vi "StatusHistory Example.vi"() -> ()   [LabVIEW 2015]
doc: "This QControl modifies a string control to display a running status history to the user. Colors are used to match the string background to give a fade-out effect.\n\n1. Click Run.\n2. Every one second an item is added to the history.\n3. Change Options to see different configurations.\n (Normally these would be set on initialize and not change. However, \n they are changable at run-time.)\n4. Click Stop to end program.\n<b> </b> <b> </b>\n©2016 Q Software Innovations, LLC (QSI)\nwritten by Quentin Alldredge\nproduced in LabVIEW 2015\n\nsupport@qsoftwareinnovations.com\nwww.qsoftwareinnovations.com\n\nAll rights reserved.\n\nRedistribution and use in source and binary forms, with or without modification, are permitted provided that the following conditions are met:\n\n * Redistributions of source code must retain the above copyright notice, this list of conditions and the following disclaimer.\n * Redistributions in binary form must reproduce the above copyright notice, this list of conditions and the following disclaimer in the documentation and/or other materials provided with the distribution.\n * Neither the name of Q Software Innovations, LLC. nor the names of its contributors may be used to endorse or promote products derived from this software without specific prior written permission.\n\nTHIS SOFTWARE IS PROVIDED BY THE COPYRIGHT HOLDERS AND CONTRIBUTORS \"AS IS\" AND ANY EXPRESS OR IMPLIED WARRANTIES, INCLUDING, BUT NOT LIMITED TO, THE IMPLIED WARRANTIES OF MERCHANTABILITY AND FITNESS FOR A PARTICULAR PURPOSE ARE DISCLAIMED. IN NO EVENT SHALL THE COPYRIGHT OWNER OR CONTRIBUTORS BE LIABLE FOR ANY DIRECT, INDIRECT, INCIDENTAL, SPECIAL, EXEMPLARY, OR CONSEQUENTIAL DAMAGES (INCLUDING, BUT NOT LIMITED TO, PROCUREMENT OF SUBSTITUTE GOODS OR SERVICES; LOSS OF USE, DATA, OR PROFITS; OR BUSINESS INTERRUPTION) HOWEVER CAUSED AND ON ANY THEORY OF LIABILITY, WHETHER IN CONTRACT, STRICT LIABILITY, OR TORT (INCLUDING NEGLIGENCE OR OTHERWISE) ARISING IN ANY WAY OUT OF THE USE OF THIS SOFTWARE, EVEN IF ADVISED OF THE POSSIBILITY OF SUCH DAMAGE."
uses:
  QControl Classes/StatusHistory/StatusHistory.lvclass
  QControl Classes/StatusHistory/Direction.ctl
panel:
  in  "Most Recent Color":u32(colorbox)
  in  "Least Recent Color":u32(colorbox)
  in  "History Size":u32=1 caption="History Size (1-10)" min=1 max=10 step=1
  in  "Direction":T1
  in  "Stop Button":bool
  in  "StatusHistory":string
  # "StatusHistory QControl Example\n\nThis QControl modifies a string control to display a running status history to the user.  Colors are used to match the string background to give a fade-out effect.\n\n1. Click Run.\n2. Every one second an item is added to the history.\n3. Change Options to see different configurations.\n    (Normally these would be set on initialize and not change.  However, \n     they are changable at run-time.)\n4. Click Stop to end program."
  # "Options"
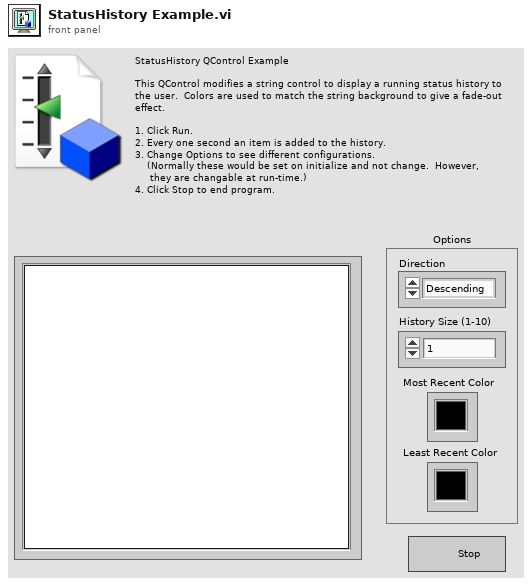
[diagram p1: front panel]
types:
  T1 = typedef "StatusHistory.lvclass/Direction.ctl" = enum16{"Descending", "Ascending"}
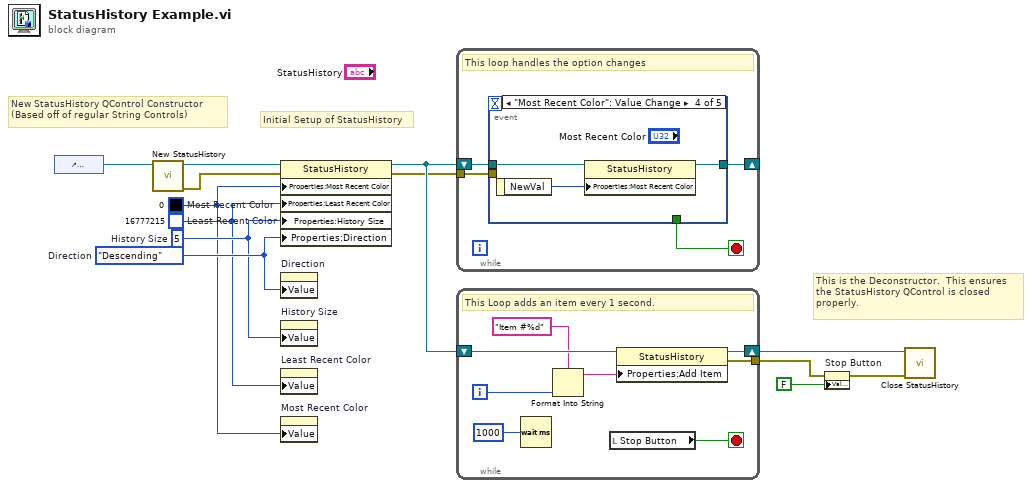
[diagram p0: block diagram]
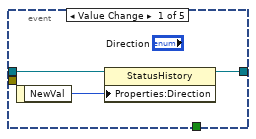
[diagram p2: hidden frame]
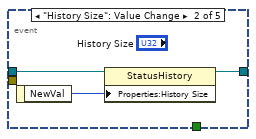
[diagram p3: hidden frame]
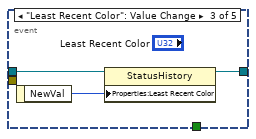
[diagram p4: hidden frame]
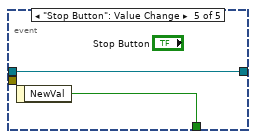
[diagram p5: hidden frame]
diagram:
  w7 = Direction."Descending"  # Direction
  w2 = u32 16777215  # Least Recent Color
  w1 = u32 0  # Most Recent Color
  w6 = u32 5  # History Size
  # "This is the Deconstructor.  This ensures \nthe StatusHistory QControl is closed \nproperly."
  # "Initial Setup of StatusHistory"
  # "New StatusHistory QControl Constructor\n(Based off of regular String Controls)"
  n1 = control-ref of="StatusHistory"() -> (w13:refnum<vi>)
  n2 = call "New StatusHistory.vi"("Reference"=w13) -> ("error out"=w11:errorcluster, "StatusHistory out"=w12:refnum<class "StatusHistory.lvclass">)  [unwired: 9 in]
  n3 = property class="StatusHistory"(reference=w12, error in=w11, "Properties:Most Recent Color"=w1, "Properties:Least Recent Color"=w2, "Properties:History Size"=w6, "Properties:Direction"=w7) -> (reference out=w10:refnum<class "StatusHistory.lvclass">, error out=w5:errorcluster)
  n4 = property on="Direction" class="Enum (strict)"("Value"=w7) -> ()  [unwired: 2 in, 2 out]
  n5 = property on="History Size" class="DigNum (strict)"("Value"=w6) -> ()  [unwired: 2 in, 2 out]
  n6 = property on="Least Recent Color" class="ColBox"("Value"=w2) -> ()  [unwired: 2 in, 2 out]
  n7 = property on="Most Recent Color" class="ColBox"("Value"=w1) -> ()  [unwired: 2 in, 2 out]
  n8 = while {
    shift-right: [w16] -> _
    shift-left: w10 -> [w17]
    tunnel: w5 -> [w14]
    stop <- w15 stop-if-true
    # "This loop handles the option changes"
    n9 = event shown="[3] \"Most Recent Color\": Value Change" {
      selector: _ -> [_ _ _ _ _]
      dyn-events: _ -> [_ _ _ _ _]
      timeout: _ -> [_ _ _ _ _]
      tunnel: w17 -> [w20 w23 w26 w29 w31]
      tunnel: [w18 w22 w25 w28 w31] -> w16
      tunnel: [_ _ _ _ w30] -> w15
      tunnel: w14 -> [_ _ _ _ _]
      event Value Change {
        n10 = event-data() -> ("NewVal"=w19:T1)  [unwired: 1 in]
        n11 = property class="StatusHistory"(reference=w20, "Properties:Direction"=w19) -> (reference out=w18:refnum<class "StatusHistory.lvclass">)  [unwired: 1 in, 1 out]
      }
      event "History Size": Value Change {
        n12 = event-data() -> ("NewVal"=w21:u32)  [unwired: 1 in]
        n13 = property class="StatusHistory"(reference=w23, "Properties:History Size"=w21) -> (reference out=w22:refnum<class "StatusHistory.lvclass">)  [unwired: 1 in, 1 out]
      }
      event "Least Recent Color": Value Change {
        n14 = event-data() -> ("NewVal"=w24:u32)  [unwired: 1 in]
        n15 = property class="StatusHistory"(reference=w26, "Properties:Least Recent Color"=w24) -> (reference out=w25:refnum<class "StatusHistory.lvclass">)  [unwired: 1 in, 1 out]
      }
      event "Most Recent Color": Value Change {
        n16 = event-data() -> ("NewVal"=w27:u32)  [unwired: 1 in]
        n17 = property class="StatusHistory"(reference=w29, "Properties:Most Recent Color"=w27) -> (reference out=w28:refnum<class "StatusHistory.lvclass">)  [unwired: 1 in, 1 out]
      }
      event "Stop Button": Value Change {
        n18 = event-data() -> ("NewVal"=w30:bool)  [unwired: 1 in]
      }
    }
  }
  n19 = while {
    shift-right: [w38] -> w4
    shift-left: w10 -> [w39]
    tunnel: [w35] -> w3
    i -> [w34]
    stop <- w36 stop-if-true
    # "This Loop adds an item every 1 second."
    n20 = Wait (ms)(milliseconds to wait=u32 1000) -> ()  [unwired: 1 out]
    n21 = Format Into String(format string="Item #%d", w34) -> (resulting string=w33:string)  [unwired: 2 in, 1 out]
    n22 = local read "Stop Button"() -> (w36:bool)
    n23 = property class="StatusHistory"(reference=w39, "Properties:Add Item"=w33) -> (reference out=w38:refnum<class "StatusHistory.lvclass">, error out=w35:errorcluster)  [unwired: 1 in]
  }
  n24 = property on="Stop Button" class="Bool (strict)"(error in=w3, "Value"=FALSE) -> (error out=w9:errorcluster)  [unwired: 1 in, 1 out]
  n25 = call "Close StatusHistory.vi"("error in (no error)"=w9, "StatusHistory in"=w4) -> ()  [unwired: 9 in, 1 out]
